vi "collect pulses.vi"(8 "error in (no error)":errorcluster, 9 "max number of pulses to show":dbl, 10 "time range":cluster{dbl, dbl}(slide)={9.216589861751153, 78525345.62211981} scale=0.0..50.0 scale format="%#_6p sec", 11 "secnario config":T1 {"mode" scale=0.0..2.0; "RF gain" min=0 max=31 step=1; "niUsrpRio Session (out)"."Daughterboard Clock Rate" format="%#.3pHz"; "niUsrpRio Session (out)"."FPGA Data Clock Rate" format="%#.3pHz"; "niUsrpRio Session (out)"."Data Clock Rate" format="%#.3pHz"; "niUsrpRio Session (out)"."Characterization Data"."Frequencies [Hz]" format="%#_6p"; "niUsrpRio Session (out)"."EEPROM Characterization Header"."Pointer to Device Data Header" format="%x"; "niUsrpRio Session (out)"."EEPROM Characterization Header"."Checksum" format="%x"; "niUsrpRio Session (out)"."Device Data Header"."Pointer to Characterization Data" format="%x"; "niUsrpRio Session (out)"."Device Data Header"."Checksum" format="%x"; "niUsrpRio Session (out)"."EEPROM Header"."Pointer to User Header" format="%x"; "niUsrpRio Session (out)"."EEPROM Header"."Pointer to Factory Header" format="%x"; "niUsrpRio Session (out)"."EEPROM Header"."Product Code" format="%x"; "niUsrpRio Session (out)"."EEPROM Header"."Checksum" format="%x"; "center frequency (Hz)" format="%#.8p"; "buffer size" step=512}) -> (0 "error out":errorcluster, 2 "PDW":cluster{"PDW":T12[], "Ton":dbl[]} {"PDW"."frequency shift" format="%#_12f"}, 3 "secnario config":T1 {"mode" scale=0.0..2.0; "RF gain" min=0 max=31 step=1; "niUsrpRio Session (out)"."Daughterboard Clock Rate" format="%#.3pHz"; "niUsrpRio Session (out)"."FPGA Data Clock Rate" format="%#.3pHz"; "niUsrpRio Session (out)"."Data Clock Rate" format="%#.3pHz"; "niUsrpRio Session (out)"."Characterization Data"."Frequencies [Hz]" format="%#_6p"; "niUsrpRio Session (out)"."EEPROM Characterization Header"."Pointer to Device Data Header" format="%x"; "niUsrpRio Session (out)"."EEPROM Characterization Header"."Checksum" format="%x"; "niUsrpRio Session (out)"."Device Data Header"."Pointer to Characterization Data" format="%x"; "niUsrpRio Session (out)"."Device Data Header"."Checksum" format="%x"; "niUsrpRio Session (out)"."EEPROM Header"."Pointer to User Header" format="%x"; "niUsrpRio Session (out)"."EEPROM Header"."Pointer to Factory Header" format="%x"; "niUsrpRio Session (out)"."EEPROM Header"."Product Code" format="%x"; "niUsrpRio Session (out)"."EEPROM Header"."Checksum" format="%x"; "center frequency (Hz)" format="%#.8p"; "buffer size" step=512})   [LabVIEW 2021]
uses:
  secnario config.ctl
  <vilib>/userdefined/High Color/nirio_resource_hc.ctl
  <instrlib>/niUsrpRio/Config/v1/Host/Public/niUsrpRio Session.ctl
  <instrlib>/_niInstr/Register Bus/v0/Host/Public/Register Bus Session.ctl
  <instrlib>/_niInstr/Register Bus/v0/Host/Private/Session Data.ctl
  <instrlib>/niUsrpRio/Config/v1/Host/Private/DB Queue Reference.ctl
  <instrlib>/niUsrpRio/Config/v1/Host/Private/Daughterboard Data.ctl
  <instrlib>/niUsrpRio/Config/v1/Host/Private/ATR state data.ctl
  <instrlib>/niUsrpRio/Config/v1/Host/Private/Antenna Configuration.ctl
  <instrlib>/niUsrpRio/Config/v1/Host/Private/CPLD Power Mode.ctl
  <instrlib>/niUsrpRio/Config/v1/Host/Public/EEPROM Header.ctl
  <instrlib>/niUsrpRio/Config/v1/Host/Public/EEPROM Device Data Header.ctl
  <instrlib>/niUsrpRio/Config/v1/Host/Public/EEPROM Characterization Header.ctl
  <instrlib>/niUsrpRio/Config/v1/Host/Public/Characterization Data.ctl
  <instrlib>/niUsrpRio/Config/v1/Host/Public/IQ Imbalance.ctl
  pdw.ctl
  mode_type.ctl
  <vilib>/Analysis/1siggen.llb/Ramp Pattern by Delta.vi
  <instrlib>/_niInstr/Basic Elements/v1/FPGA/Private/Count Up U64.vi
  <vilib>/Analysis/NI_AALBase.lvlib
  <instrlib>/_niInstr/Basic Elements/v1/FPGA/niInstr Basic Elements v1 FPGA.lvlib
  <instrlib>/_niInstr/Register Bus/v0/Host/niInstr Register Bus v0 Host.lvlib
  <instrlib>/niUsrpRio/Config/v1/Host/niUsrpRio Config v1 Host.lvlib
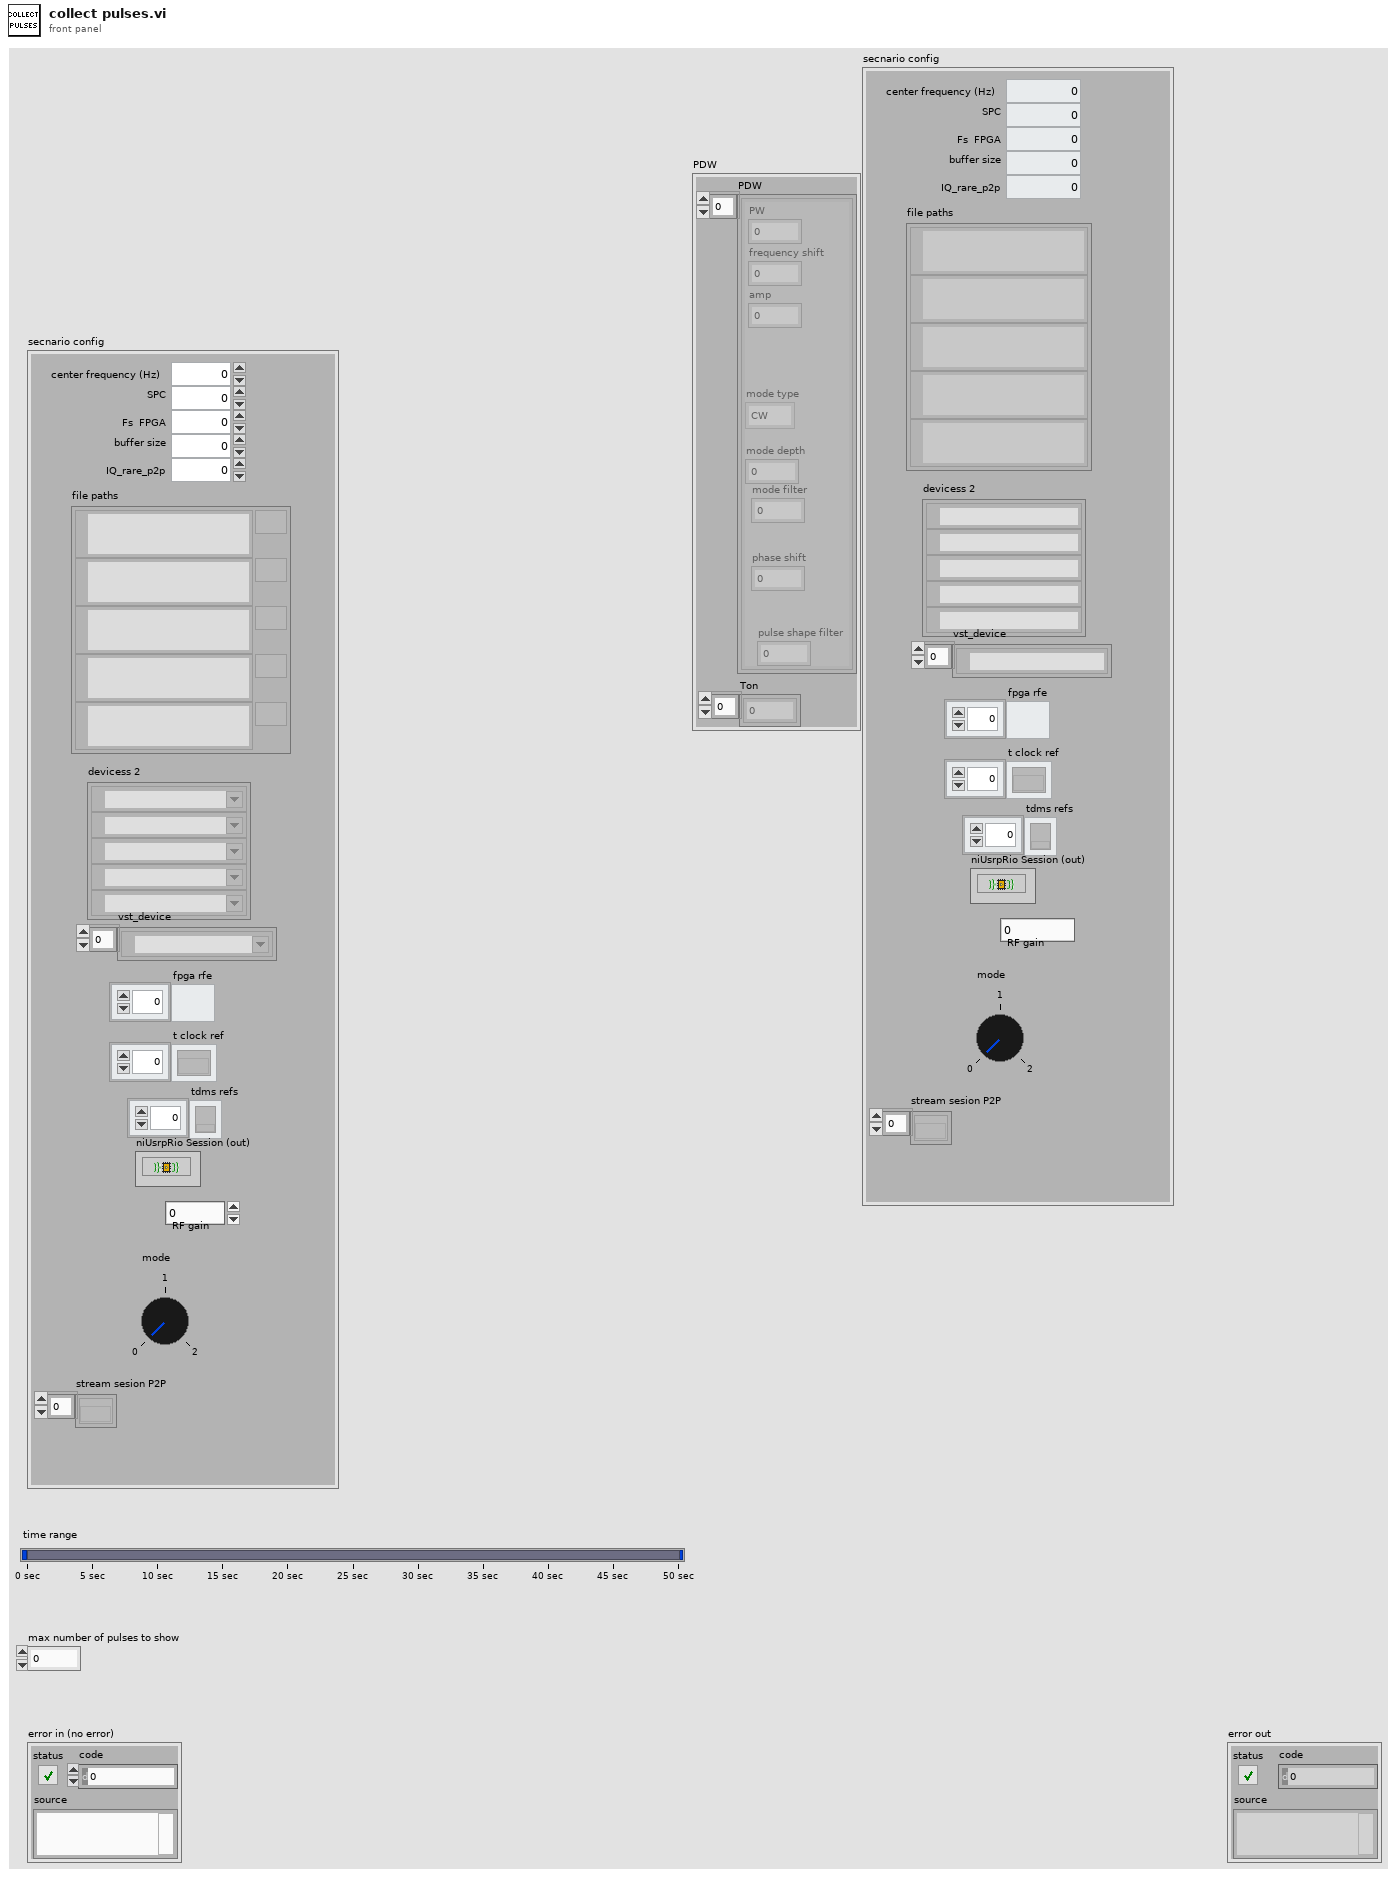
[diagram p1: front panel]
types:
  T1 = typedef "secnario config.ctl" = cluster{"devicess 2":T2[], "file paths":path[], "buffer size":u32, "Fs  FPGA":dbl, "SPC":dbl, "center frequency (Hz) ":dbl, "t clock ref":refnum<k20>[], "fpga rfe":refnum<k20>[], "tdms refs":refnum<k34>[], "niUsrpRio Session (out)":T3, "RF gain ":i32, "mode":u8, "vst_device":refnum<k15>[], "IQ_rare_p2p":dbl, "stream sesion P2P":refnum<k20>[]}
  T2 = typedef "nirio_resource_hc.ctl" = tag
  T3 = typedef "niUsrpRio Config v1 Host.lvlib/niUsrpRio Session.ctl" = cluster{"FPGA Interface":refnum<k20>, "RIO Interface Number":u32, "Data Clock Rate":u32, "FPGA Data Clock Rate":u32, "Global Settings Register Bus":T4, "Radio 0 Settings Register Bus":T4, "Radio 1 Settings Register Bus":T4, "Radio Settings Bus Semaphore":T5, "DB Queues":T6[], "Characterization Data Valid?":bool, "EEPROM Header":T7, "Device Data Header":T8, "EEPROM Characterization Header":T9, "Characterization Data":T10[], "FPGA Current Version":u32, "FPGA Oldest Compatible Version":u32, "Fixed Logic Current Version":u32, "Fixed Logic Oldest Compatible Version":u32, "FPGA Radio Settings Bus Current Version":u32, "FPGA Radio Settings Bus Oldest Compatible Version":u32, "FPGA Board Config Current Version":u32, "FPGA Board Config Oldest Compatible Version":u32, "Daughterboard Clock Rate":u32, "daughterboard configuration session handles":u64[]}
  T4 = typedef "niInstr Register Bus v0 Host.lvlib/Register Bus Session.ctl" = refnum<queue>
  T5 = typedef "Semaphore RefNum" = refnum<k1>
  T6 = typedef "niUsrpRio Config v1 Host.lvlib/DB Queue Reference.ctl" = refnum<queue>
  T7 = typedef "niUsrpRio Config v1 Host.lvlib/EEPROM Header.ctl" = cluster{"Checksum":u32, "Product Code":u16, "Hardware Current Version":u16, "Hardware Oldest Compatible Version":u16, "EEPROM Map Current Version":u16, "EEPROM Map Oldest Compatible Version":u16, "User Password":string, "Pointer to Factory Header":u32, "Pointer to User Header":u32, "Recommended Interval":u16, "Number of Reserved Bytes":i32, "Number of Daughterboards":u8, "Daughterboard IDs":u16[], "Daughterboard Serial Numbers":string[]}
  T8 = typedef "niUsrpRio Config v1 Host.lvlib/EEPROM Device Data Header.ctl" = cluster{"Checksum":u32, "Number of Channels":u8, "Number of Gain Settings":u16[], "Pointer to Characterization Data":u32[], "Number of Reserved Bytes":i32, "Number of Frequencies":u16[]}
  T9 = typedef "niUsrpRio Config v1 Host.lvlib/EEPROM Characterization Header.ctl" = cluster{"Checksum":u32, "Date":timestamp, "Temperature":sgl, "Misc. Info":string, "Pointer to Device Data Header":u32, "Number of Reserved Bytes":i32}
  T10 = typedef "niUsrpRio Config v1 Host.lvlib/Characterization Data.ctl" = cluster{"Gains[dB]":dbl[], "Frequencies [Hz]":dbl[], "IQ Imbalance Table":T11[], "Measured Gains[dB]":dbl[][]}
  T11 = typedef "niUsrpRio Config v1 Host.lvlib/IQ Imbalance.ctl" = cluster{"Gain Imbalance [linear]":dbl, "Phase Imbalance [radians]":dbl, "Offset":cdb}
  T12 = typedef "pdw.ctl" = cluster{"PW":u32, "frequency shift":fxp<+/-,48,0>, "amp":fxp<+/-,18,1>, "mode type":T13, "mode depth":u32, "mode filter":u8, "phase shift":fxp<+/-,16,1>, "pulse shape filter":u8}
  T13 = typedef "mode_type.ctl" = enum8{"CW", "NC - CW", "NC - cw", "LFM", "BPSK", "QPSK"}
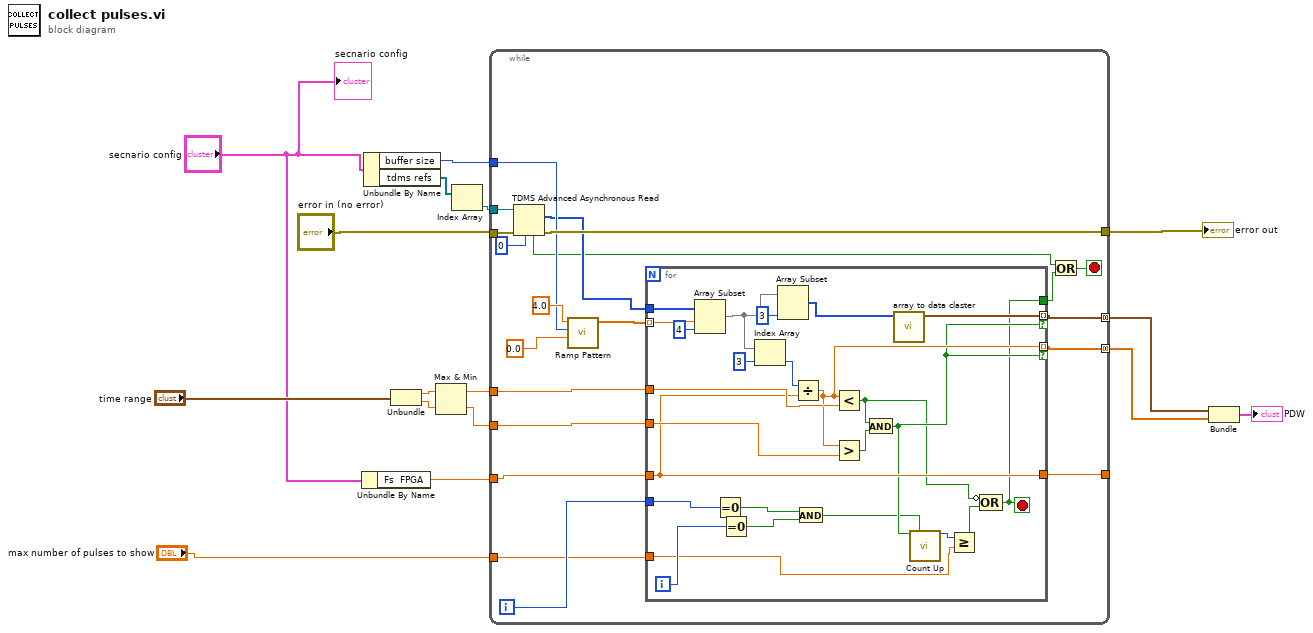
[diagram p0: block diagram]
diagram:
  n1 = Unbundle By Name("secnario config") -> ("Fs  FPGA"=w10:dbl)
  n2 = Unbundle By Name("secnario config") -> ("buffer size"=w12:u32, "tdms refs"=w14:refnum<k34>[])
  n3 = Unbundle("time range") -> (w5:dbl, w6:dbl)
  n4 = Max & Min(x=w5, y=w6) -> (max(x,y)=w9:dbl, min(x,y)=w8:dbl)
  n5 = Index Array(array=w14) -> (element=w13:refnum<k34>)  [unwired: 1 in]
  n6 = while {
    tunnel: w13 -> [w23]
    tunnel: "error in (no error)" -> [w36]
    tunnel: [w35] -> w15
    tunnel: w12 -> [w32]
    tunnel: w10 -> [w29]
    tunnel: w8 -> [w28]
    tunnel: w9 -> [w27]
    tunnel: [w26] -> w2 mode=concatenating
    tunnel: [w25] -> w3 mode=concatenating
    tunnel: [w24] -> _
    tunnel: "max number of pulses to show" -> [w17]
    i -> [w21]
    stop <- w18 stop-if-true
    n7 = TDMS Advanced Asynchronous Read(6:u64 0 ("data type"), 8:w36, 11:w23) -> (0:w35:errorcluster, 2:w30:u64[], 4:w20:bool)  [unwired: 1 out]
    n8 = call-poly <vilib>:"Ramp Pattern.vi"("start"=0.0, "end"=w32, "delta"=4.0) -> ("Ramp Pattern"=w31:dbl[])  [unwired: 6 in, 2 out]
    n9 = for {
      tunnel: w31 -> [w61] mode=indexing
      tunnel: w30 -> [w60]
      tunnel: w29 -> [w51]
      tunnel: w28 -> [w56]
      tunnel: w27 -> [w55]
      tunnel: [w53] -> w25 mode=indexing if=w47
      tunnel: [w52] -> w26 mode=indexing if=w47
      tunnel: [w51] -> w24
      tunnel: w21 -> [w42]
      tunnel: [w38] -> w19
      tunnel: w17 -> [w37]
      i -> [w43]
      stop <- w38 stop-if-true
      n10 = Array Subset(array=w60, index=w61, length=4) -> (w50:u64[])
      n11 = Equal To 0?(x=w42) -> (x = 0?=w41:bool)
      n12 = Equal To 0?(x=w43) -> (x = 0?=w40:bool)
      n13 = Index Array(array=w50, index=3) -> (element=w57:u64)
      n14 = Array Subset(array=w50, length=3) -> (w48:u64[])  [unwired: 1 in]
      n15 = Divide(x=w57, y=w51) -> (x/y=w52:dbl)
      n16 = And(x=w41, y=w40) -> (x .and. y?=w39:bool)
      n17 = Less?(x=w52, y=w55) -> (x < y?=w45:bool)
      n18 = Greater?(x=w52, y=w56) -> (0:w54:bool)
      n19 = And(x=w45, y=w54) -> (x .and. y?=w47:bool)
      n20 = call "array to data claster.vi"("Array"=w48) -> ("Cluster"=w53:T12)  [unwired: 10 in]
      n21 = call-poly <instrlib>:"Count Up.vi"("increment"=w47, "reset"=w39) -> ("count out"=w46:u64)  [unwired: 13 in]
      n22 = Greater Or Equal?(x=w46, y=w37) -> (x >= y?=w44:bool)
      n23 = Compound Arithmetic op=OR(invert w45, w44) -> (w38:bool)
    }
    n24 = Or(x=w20, y=w19) -> (x .or. y?=w18:bool)
  }
  "error out" <- w15
  n25 = Bundle(w3, w2) -> (→"PDW":cluster{T12[], dbl[]})  [unwired: 1 in]
  "secnario config" <- "secnario config"
